vi "main.vi"() -> ()   [LabVIEW 2018]
panel:
  out "First Measurment":bool
  in  "Outfile Path 2":path
  in  "Inital List":string[](array[string])
  in  "Tab Control":T1(tab)
  in  "Sampling Time (s)":u32=2
  in  "Save\n Waveform":bool
  out "Wire Length (mm)":dbl
  out "Linear Density (µg/mm)":dbl
  in  "Save FFT":bool
  in  "sMDT Code":string
  in  "Charge Time (s)":dbl=1.0
  out "Waveform":waveform(dbl)(graph)
  out "FFT":waveform(dbl)(graph)
  out "Charge time(s)":dbl caption="Elapsed Time (s)"
  out "Nth Measurement":i32
  out "DAQ Output (V)":dbl
  out "Tension (g)":dbl format="%#.2f"
  out "Frequency(Hz)":dbl
  in  "User ID":i32(ring) items=["Kyle", "Henry", "Victor", "Dravin", "Braden", "Jake", "Jason", "Akshit", "Jaime", "Mike"]
  out "Charging ?":bool
  in  "Get Tension":bool
  out "Tension Error (g)":dbl format="%#.2g"
  out "Wire Length (mm)":dbl
  out "Linear Density (µg/mm)":dbl
  in  "File Format":enum32{"BMP", "EPS", "EMF", "PICT"}(ring)
  in  "Save Live \nWaveform":bool
  in  "File Format":enum32{"BMP", "EPS", "EMF", "PICT"}(ring)
  out "Live \nWaveform":waveform(dbl)(graph)
  in  "Save Live FFT":bool
  in  "File Format":enum32{"BMP", "EPS", "EMF", "PICT"}(ring)
  out "Live FFT":waveform(dbl)(graph)
  in  "Save Last \nWaveform":bool
  in  "File Format":enum32{"BMP", "EPS", "EMF", "PICT"}(ring)
  out "Last \nWaveform":waveform(dbl)(graph)
  in  "Save Last FFT":bool
  in  "File Format":enum32{"BMP", "EPS", "EMF", "PICT"}(ring)
  out "Last FFT":waveform(dbl)(graph)
  out "Measurements":string[][](array[string])
  in  "Calibration Factor":dbl=1.0
  in  "Frequency Error (Hz)":dbl
  in  "Wire Linear Density Error (µg/mm)":dbl=0.05
  in  "Wire Length Error (mm)":dbl=0.1
  out "User List":string[](array[string])
  in  "Remove":bool
  in  "Add":bool
  in  "User ID":string
  in  "User List File":path
  in  "Wire Linear Density (µg/mm)":dbl=38.8
  # "ATLAS Phase II sMDT Wire Tension Test"
  # "User Controls"
  # "Status"
  # "sMDT Length"
  # "Waveform From Wire"
  # "Measurements"
  # "Spectral Decomposition (FFT)"
  # "Live Wavefrom from Wire"
  # "Live Spectral Decomposition (FFT)"
  # "Last Wavefrom from Wire"
  # "Last Spectral Decomposition (FFT)"
  # "Measurements"
  # "User ID"
  # "Date / Time"
  # "sMDT Code"
  # "Wire Length"
  # "Linear Density"
  # "Frequency"
  # "Tension/g"
  # "Tension/g Error"
  # "Add/Remove Users"
  # "Set Physical Constants"
  # "Calibration"
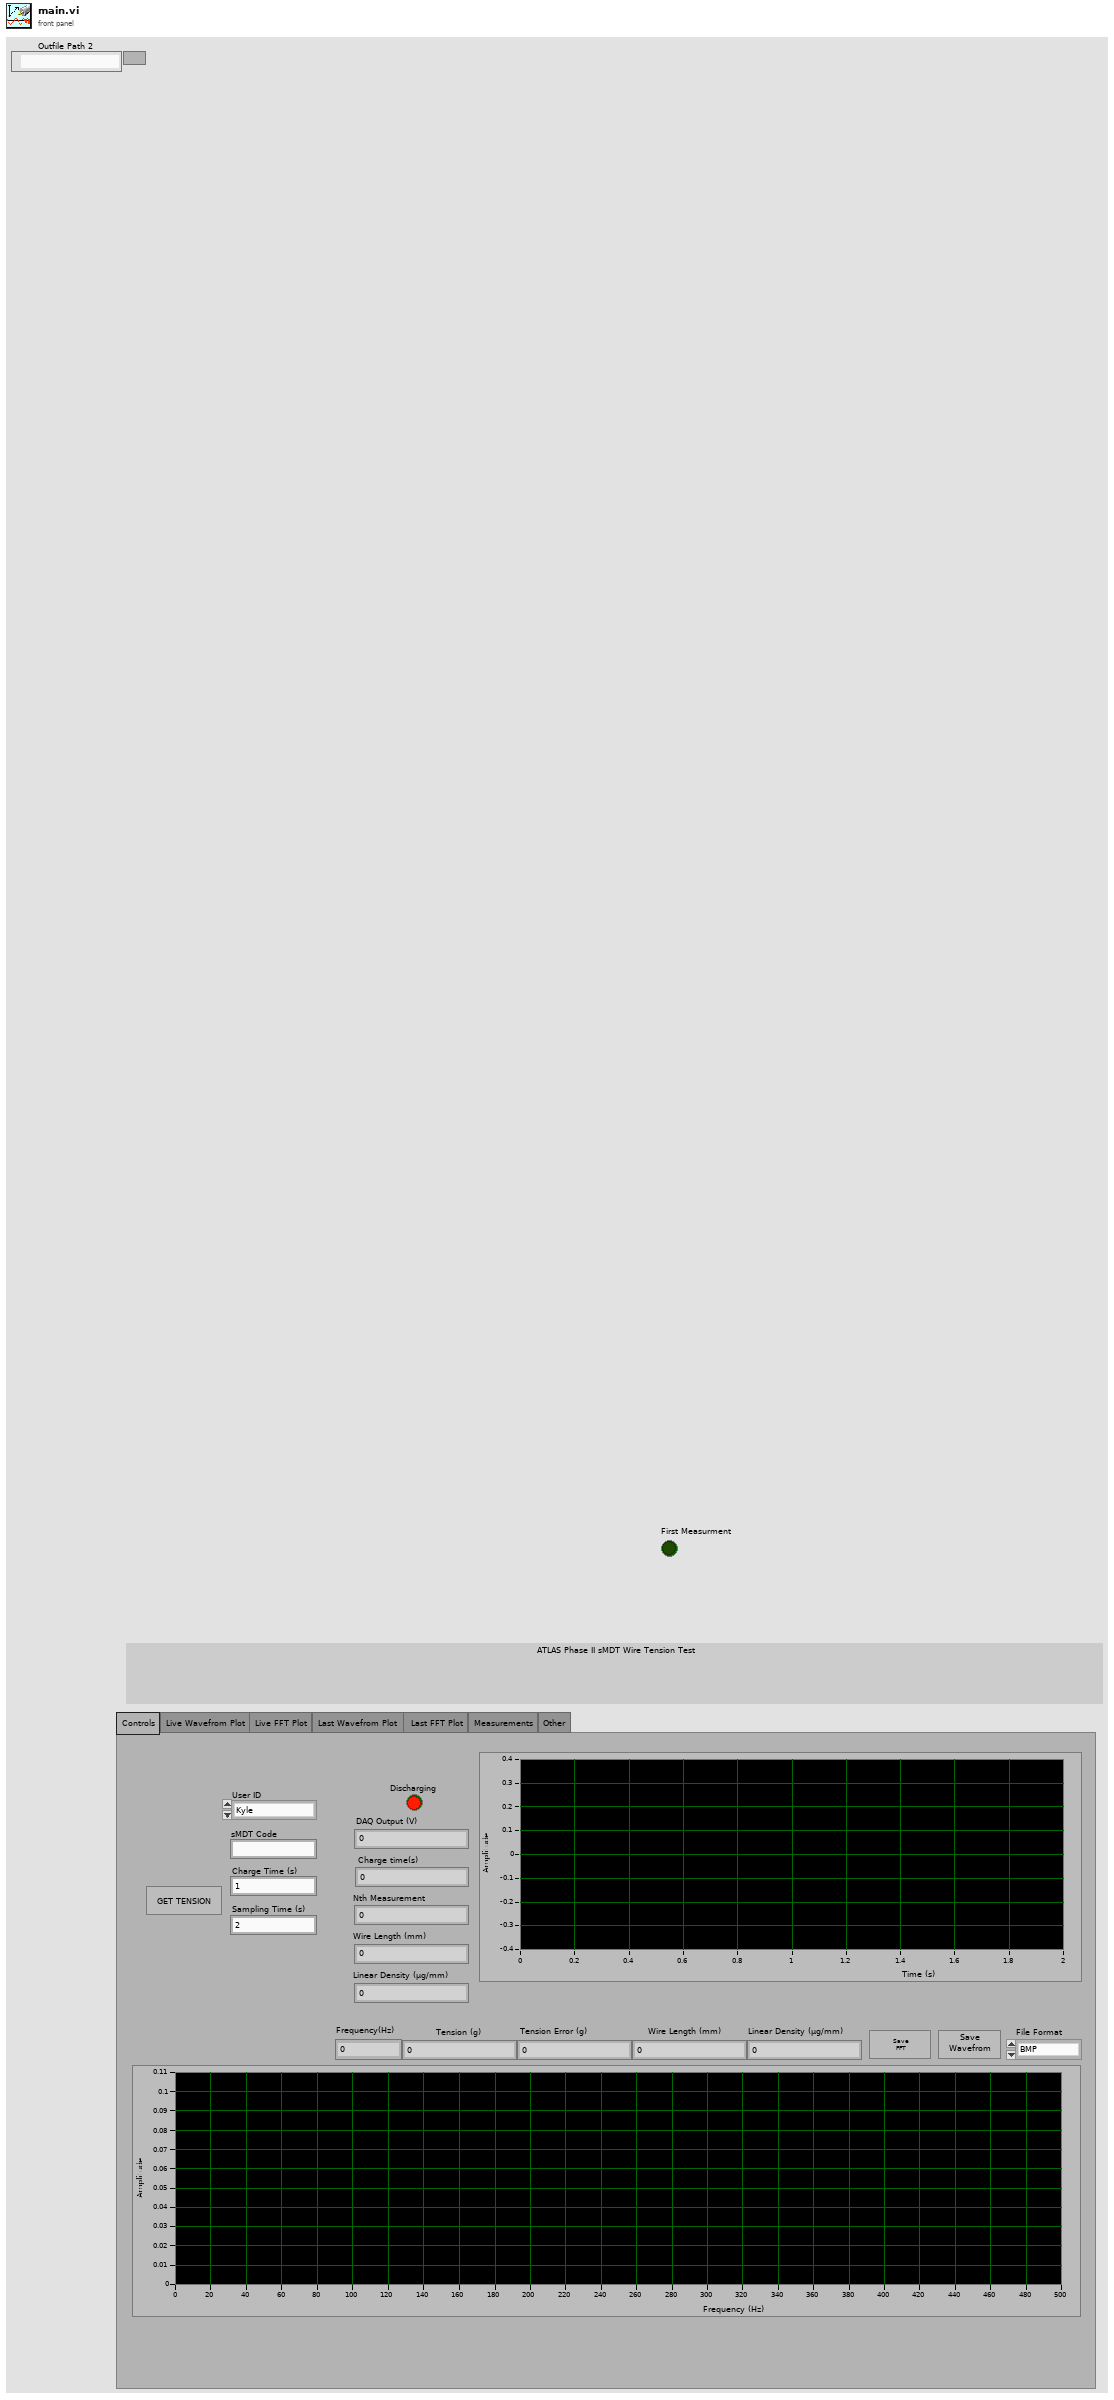
[diagram p1: front panel]
types:
  T1 = enum32{"Controls", "Live Wavefrom Plot", "Live FFT Plot", "Last Wavefrom Plot ", "Last FFT Plot ", "Measurements", "Other"}
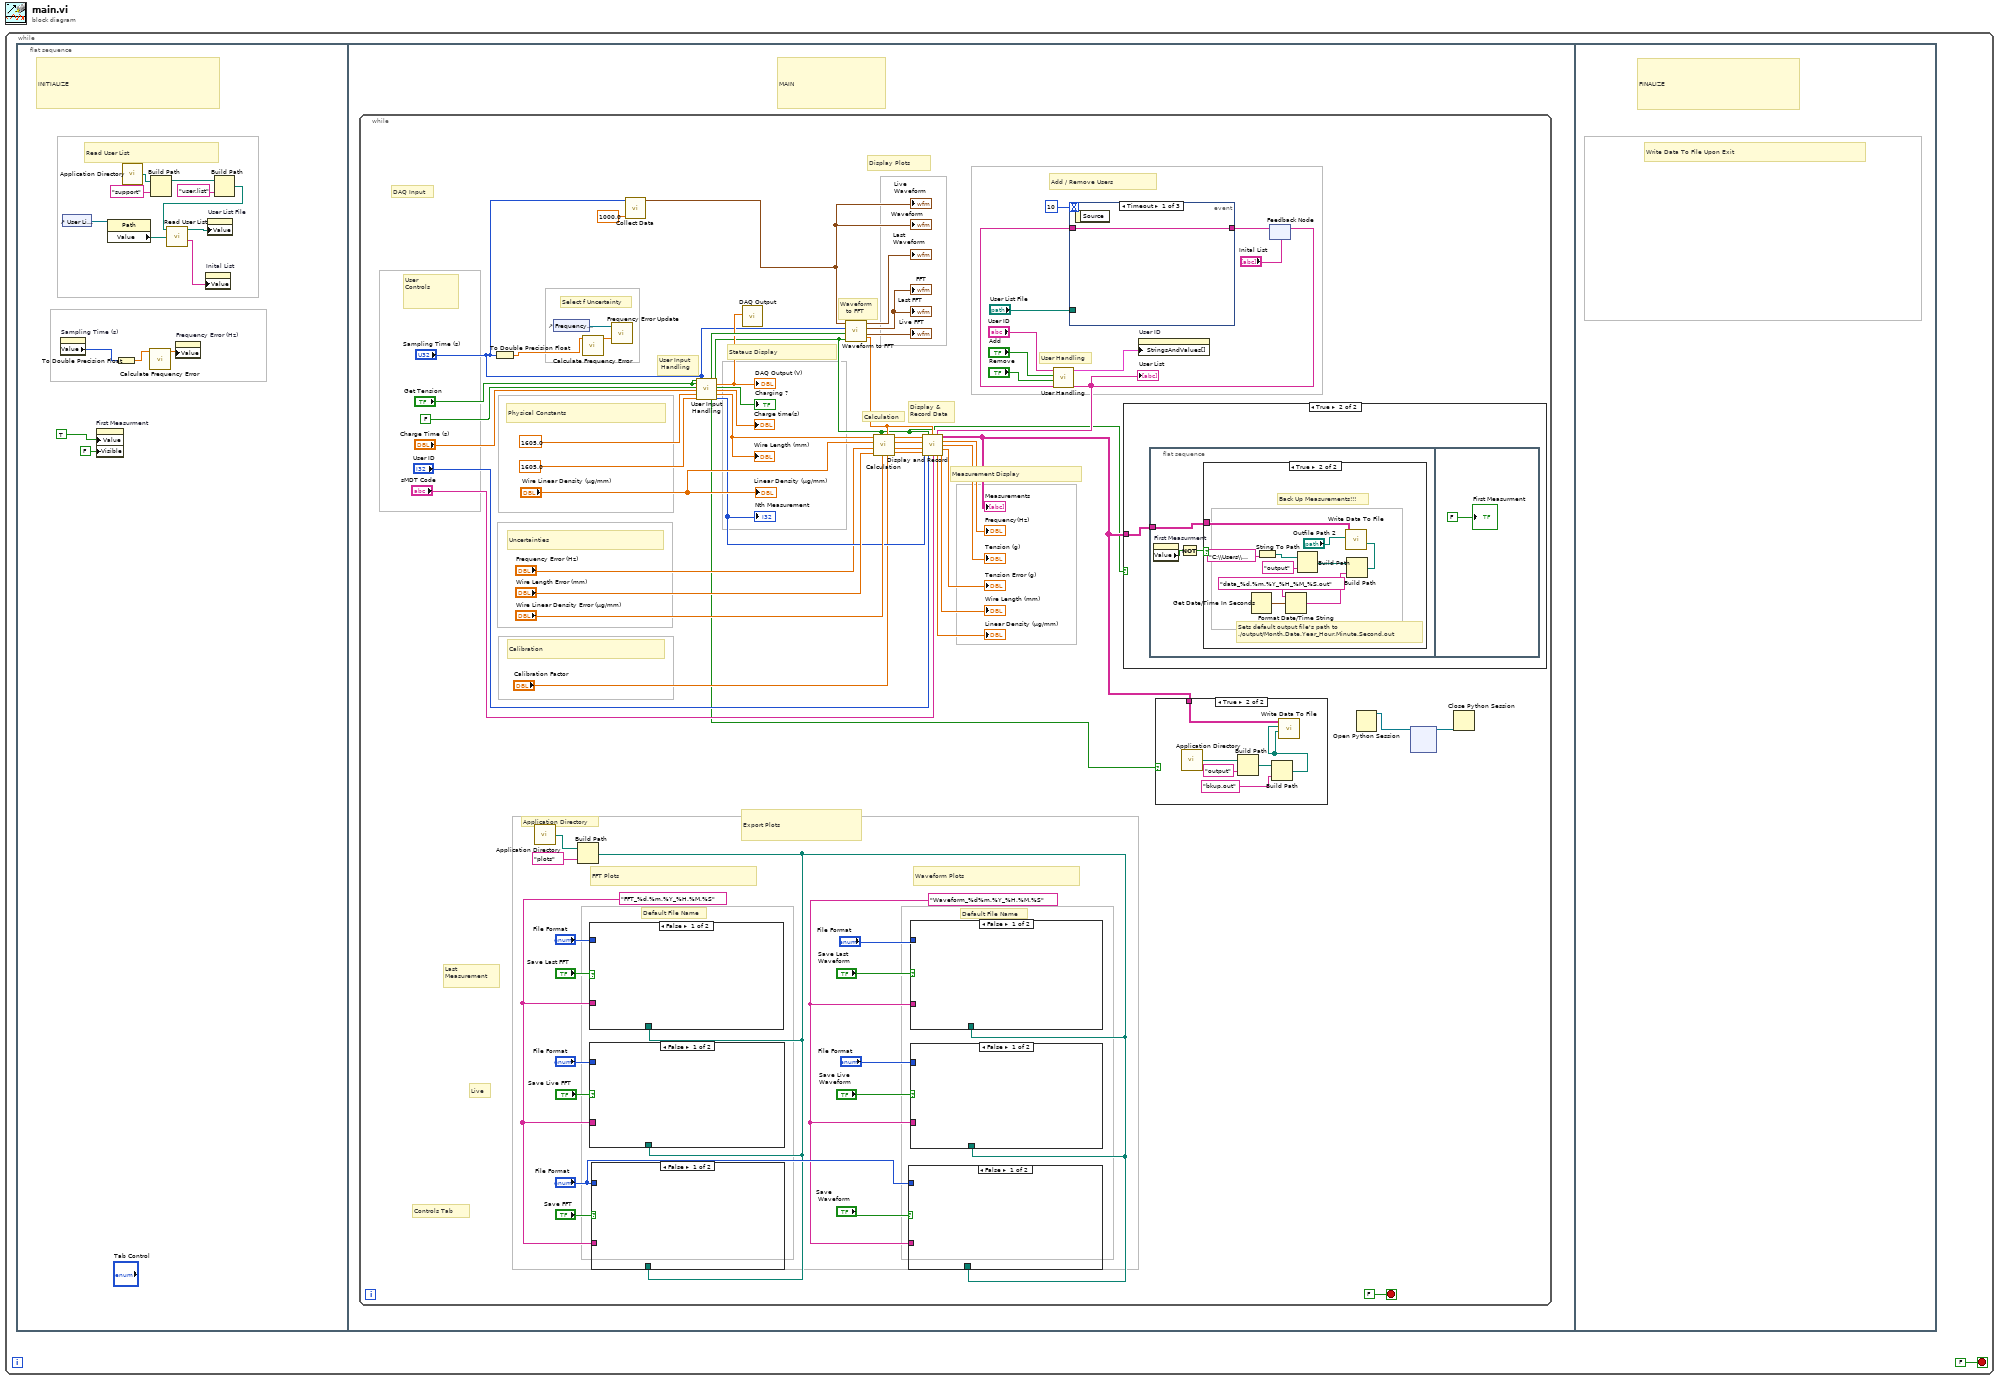
[diagram p0: block diagram]
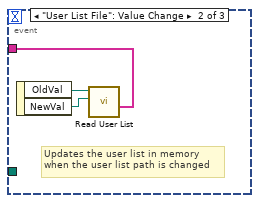
[diagram p5: hidden frame]
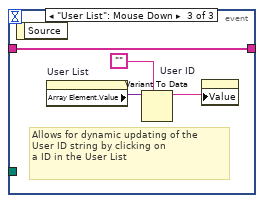
[diagram p6: hidden frame]
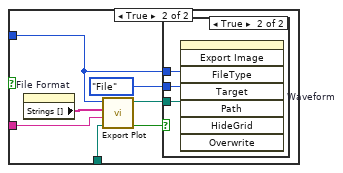
[diagram p7: hidden frame]
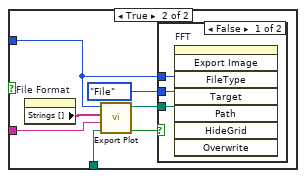
[diagram p9: hidden frame]
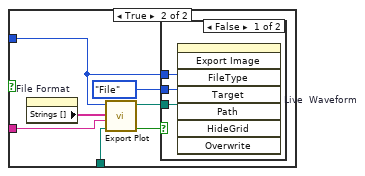
[diagram p11: hidden frame]
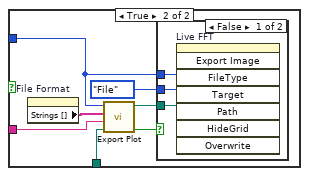
[diagram p13: hidden frame]
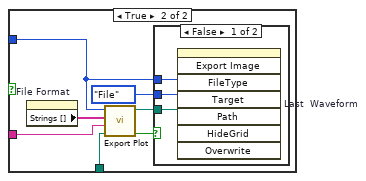
[diagram p15: hidden frame]
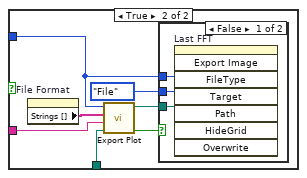
[diagram p17: hidden frame]
diagram:
  n1 = while {
    stop <- FALSE stop-if-true
    n2 = flat-sequence {
      frame #0 {
        # "INITIALIZE"
        # "Read User List"
        n3 = property on="Sampling Time (s)" class="DigNum (strict)"() -> ("Value"=w6:u32)  [unwired: 2 in, 2 out]
        n4 = control-ref of="User List File"() -> (w8:refnum<vi>)
        n5 = property on="First Measurment" class="Bool (strict)"("Value"=TRUE ("First Measurment"), "Visible"=FALSE) -> ()  [unwired: 2 in, 2 out]
        n6 = property on="Property Node" class="Path"(reference=w8) -> ("Value"=w14:path)  [unwired: 1 in, 2 out]
        n7 = To Double Precision Float(number=w6) -> (double precision float=w4:dbl)
        n8 = call <vilib>:"Application Directory.vi"() -> ("Application Directory"=w10:path)
        n9 = call "Calculate Frequency Error.vi"("Sampling Time"=w4) -> ("df"=w5:dbl)  [unwired: 10 in]
        n10 = Build Path(base path=w10, name or relative path="support") -> (appended path=w13:path)
        n11 = property on="Frequency Error (Hz)" class="DigNum (strict)"("Value"=w5) -> ()  [unwired: 2 in, 2 out]
        n12 = Build Path(base path=w13, name or relative path="user.list") -> (appended path=w15:path)
        n13 = call "Read User List.vi"("User List File"=w14, "User List File Default"=w15) -> ("Array"=w9:string[], "Path Out"=w7:path)  [unwired: 8 in]
        n14 = property on="Inital List" class="Arr (strict)"("Value"=w9) -> ()  [unwired: 2 in, 2 out]
        n15 = property on="User List File" class="Path"("Value"=w7) -> ()  [unwired: 2 in, 2 out]
      }
      frame #1 {
        # "MAIN"
        n16 = while {
          stop <- FALSE stop-if-true
          w63 = "Waveform_%d%m.%Y_%H.%M.%S"
          w64 = "FFT_%d.%m.%Y_%H.%M.%S"
          # "User Handling"
          # "Calibration"
          # "Select f Uncertainty"
          # "User Input \n Handling"
          # "Export Plots"
          # "Controls Tab"
          # "Live"
          # "Last \nMeasurement"
          # "Application Directory"
          # "Display Plots"
          # "Default File Name"
          # "Default File Name"
          # "DAQ Input"
          # "Measurement Display"
          # "Stataus Display"
          # "Display &\nRecord Data"
          # "Calculation"
          # "Waveform\n   to FFT"
          # "Waveform Plots"
          # "Uncertainties"
          # "Physical Constants"
          # "FFT Plots"
          # "Add / Remove Users"
          # "User \nControls"
          n17 = To Double Precision Float(number="Sampling Time (s)") -> (double precision float=w30:dbl)
          n18 = call <vilib>:"Application Directory.vi"() -> ("Application Directory"=w35:path)
          n19 = control-ref of="Frequency Error (Hz)"() -> (w37:refnum<vi>)
          n20 = Build Path(base path=w35, name or relative path="plots") -> (appended path=w34:path)
          n21 = call "Calculate Frequency Error.vi"("Sampling Time"=w30) -> ("df"=w31:dbl)  [unwired: 10 in]
          n22 = case shown="False" "Save Last FFT" {
            tunnel: "File Format" -> [_ w164]
            tunnel: w64 -> [_ w170]
            tunnel: w34 -> [_ w169]
            frame False {
            }
            frame True {
              n23 = property on="File Format" class="Enum (strict)"() -> ("Strings []"=w168:string[])  [unwired: 2 in, 2 out]
              n24 = call "Export Plot.vi"("Path 2"=w169, "String"=w170, "Array"=w168, "File Format"=w164) -> ("Canceled?"=w167:bool, "Path"=w166:path)  [unwired: 6 in]
              n25 = case shown="False" w167 {
                tunnel: w166 -> [w173 _]
                tunnel: enum32{"File", "Clipboard"}."File" ("Target") -> [w172 _]
                tunnel: w164 -> [w171 _]
                frame False {
                  n26 = invoke on="Last FFT" class="WFGraph (strict)" method="Export Image"("FileType"=w171, "Target"=w172, "Path"=w173) -> ()  [unwired: 5 in, 8 out]
                }
                frame True {
                }
              }
            }
          }
          n27 = case shown="False" "Save Live FFT" {
            tunnel: w64 -> [_ w150]
            tunnel: w34 -> [_ w149]
            tunnel: "File Format" -> [_ w146]
            frame False {
            }
            frame True {
              n28 = property on="File Format" class="Enum (strict)"() -> ("Strings []"=w145:string[])  [unwired: 2 in, 2 out]
              n29 = call "Export Plot.vi"("Path 2"=w149, "String"=w150, "Array"=w145, "File Format"=w146) -> ("Canceled?"=w144:bool, "Path"=w148:path)  [unwired: 6 in]
              n30 = case shown="False" w144 {
                tunnel: w148 -> [w153 _]
                tunnel: enum32{"File", "Clipboard"}."File" ("Target") -> [w152 _]
                tunnel: w146 -> [w151 _]
                frame False {
                  n31 = invoke on="Live FFT" class="WFGraph (strict)" method="Export Image"("FileType"=w151, "Target"=w152, "Path"=w153) -> ()  [unwired: 5 in, 8 out]
                }
                frame True {
                }
              }
            }
          }
          n32 = case shown="False" "Save FFT" {
            tunnel: "File Format" -> [_ w126]
            tunnel: w64 -> [_ w130]
            tunnel: w34 -> [_ w129]
            frame False {
            }
            frame True {
              n33 = property on="File Format" class="Enum (strict)"() -> ("Strings []"=w125:string[])  [unwired: 2 in, 2 out]
              n34 = call "Export Plot.vi"("Path 2"=w129, "String"=w130, "Array"=w125, "File Format"=w126) -> ("Canceled?"=w124:bool, "Path"=w128:path)  [unwired: 6 in]
              n35 = case shown="False" w124 {
                tunnel: w128 -> [w133 _]
                tunnel: enum32{"File", "Clipboard"}."File" ("Target") -> [w132 _]
                tunnel: w126 -> [w131 _]
                frame False {
                  n36 = invoke on="FFT" class="WFGraph (strict)" method="Export Image"("FileType"=w131, "Target"=w132, "Path"=w133) -> ()  [unwired: 5 in, 8 out]
                }
                frame True {
                }
              }
            }
          }
          n37 = call "Frequency Error Update.vi"("Source"=w31, "Target"=w37) -> ()  [unwired: 10 in]
          n38 = call "Collect Data.vi"("rate"=1000.0, "sample time"="Sampling Time (s)") -> ("Waveform"=w28:waveform(dbl))  [unwired: 9 in]
          "Waveform" <- w28
          "Live \nWaveform" <- w28
          n39 = call "User Input Handling.vi"("Record?"="Get Tension", "Get Tension"="Get Tension", "Short"=FALSE, "Charge Time (s)"="Charge Time (s)", "Short Wire Length (mm)"=1605.0, "Long Wire Length (mm)"=1605.0, "Sampling Time (s)"="Sampling Time (s)") -> ("Has measured?"=w48:bool, "Made Measurement?"=w22:bool, "t < X ?"=w18:bool, "DAQ"=w29:dbl, "charging"=→"Charging ?":bool, "Elapsed time(s)"=→"Charge time(s)":dbl, "Wire Length Out"=w54:dbl, "Nth Measurement"=w49:i32)  [unwired: 5 in]
          "Nth Measurement" <- w49
          "DAQ Output (V)" <- w29
          "Wire Length (mm)" <- w54
          n40 = call "DAQ Output.vi"("Numeric"=w29) -> ()  [unwired: 11 in]
          n41 = call "Waveform to FFT.vi"("t < X ?"=w18, "Measured?"=w48, "Sampling Time(s)"="Sampling Time (s)", "Waveform in"=w28) -> ("FFT out"=→"Live FFT":waveform(dbl), "Last FFT"=→"FFT" →"Last FFT":waveform(dbl), "Last Waveform"=→"Last \nWaveform":waveform(dbl), "Frequency"=w62:dbl)  [unwired: 4 in]
          n42 = call "Calculation.vi"("Calibration Factor"="Calibration Factor", "Frequency (Hz)"=w62, "dµ (µg/mm)"="Wire Linear Density Error (µg/mm)", "t < 1.5 s ?"=w18, "dL (mm)"="Wire Length Error (mm)", "df (Hz)"="Frequency Error (Hz)", "Wire Linear Density In"="Wire Linear Density (µg/mm)", "Wire Length In"=w54) -> ("Linear Density (µm/mm)"=w77:dbl, "Wire Length (mm)"=w76:dbl, "dT (g)"=w75:dbl, "Tension (g)"=w78:dbl)
          n43 = case shown="False" "Save\n Waveform" {
            tunnel: "File Format" -> [_ w117]
            tunnel: w63 -> [_ w120]
            tunnel: w34 -> [_ w119]
            frame False {
            }
            frame True {
              n44 = property on="File Format" class="Enum (strict)"() -> ("Strings []"=w115:string[])  [unwired: 2 in, 2 out]
              n45 = call "Export Plot.vi"("Path 2"=w119, "String"=w120, "Array"=w115, "File Format"=w117) -> ("Canceled?"=w114:bool, "Path"=w118:path)  [unwired: 6 in]
              n46 = case shown="True" w114 {
                tunnel: w118 -> [_ w123]
                tunnel: w117 -> [_ w122]
                tunnel: enum32{"File", "Clipboard"}."File" ("Target") -> [_ w121]
                frame False {
                }
                frame True {
                  n47 = invoke on="Waveform" class="WFGraph (strict)" method="Export Image"("FileType"=w122, "Target"=w121, "Path"=w123) -> ()  [unwired: 5 in, 8 out]
                }
              }
            }
          }
          n48 = case shown="False" "Save Last \nWaveform" {
            tunnel: "File Format" -> [_ w156]
            tunnel: w63 -> [_ w160]
            tunnel: w34 -> [_ w159]
            frame False {
            }
            frame True {
              n49 = property on="File Format" class="Enum (strict)"() -> ("Strings []"=w155:string[])  [unwired: 2 in, 2 out]
              n50 = call "Export Plot.vi"("Path 2"=w159, "String"=w160, "Array"=w155, "File Format"=w156) -> ("Canceled?"=w154:bool, "Path"=w158:path)  [unwired: 6 in]
              n51 = case shown="False" w154 {
                tunnel: w158 -> [w163 _]
                tunnel: enum32{"File", "Clipboard"}."File" ("Target") -> [w162 _]
                tunnel: w156 -> [w161 _]
                frame False {
                  n52 = invoke on="Last  Waveform" class="WFGraph (strict)" method="Export Image"("FileType"=w161, "Target"=w162, "Path"=w163) -> ()  [unwired: 5 in, 8 out]
                }
                frame True {
                }
              }
            }
          }
          n53 = case shown="False" "Save Live \nWaveform" {
            tunnel: w63 -> [_ w140]
            tunnel: "File Format" -> [_ w137]
            tunnel: w34 -> [_ w135]
            frame False {
            }
            frame True {
              n54 = property on="File Format" class="Enum (strict)"() -> ("Strings []"=w136:string[])  [unwired: 2 in, 2 out]
              n55 = call "Export Plot.vi"("Path 2"=w135, "String"=w140, "Array"=w136, "File Format"=w137) -> ("Canceled?"=w134:bool, "Path"=w138:path)  [unwired: 6 in]
              n56 = case shown="False" w134 {
                tunnel: enum32{"File", "Clipboard"}."File" ("Target") -> [w143 _]
                tunnel: w138 -> [w142 _]
                tunnel: w137 -> [w141 _]
                frame False {
                  n57 = invoke on="Live  Waveform" class="WFGraph (strict)" method="Export Image"("FileType"=w141, "Target"=w143, "Path"=w142) -> ()  [unwired: 5 in, 8 out]
                }
                frame True {
                }
              }
            }
          }
          n58 = feedback #1("Inital List") -> (w38:string[])
          n59 = event shown="[0] Timeout" {
            selector: _ -> [_ _ _]
            dyn-events: _ -> [_ _ _]
            timeout: 10 -> [_ _ _]
            tunnel: [w106 w107 w110] -> w45
            tunnel: w38 -> [w106 _ w110]
            tunnel: "User List File" -> [_ _ _]
            event Timeout {
              n60 = event-data() -> ()  [unwired: 1 in, 1 out]
            }
            event "User List File": Value Change {
              # "Updates the user list in memory\nwhen the user list path is changed"
              n61 = event-data() -> ("OldVal"=w109:path, "NewVal"=w108:path)  [unwired: 1 in]
              n62 = call "Read User List.vi"("User List File"=w108, "User List File Default"=w109) -> ("Array"=w107:string[])  [unwired: 8 in, 1 out]
            }
            event "User List": Mouse Down {
              # "Allows for dynamic updating of the \nUser ID string by clicking on \na ID in the User List"
              n63 = event-data() -> ()  [unwired: 1 in, 1 out]
              n64 = property on="User List" class="Arr (strict)"() -> ("Array Element.Value"=w111:variant)  [unwired: 2 in, 2 out]
              n65 = Variant To Data(type="", Variant=w111) -> (data=w112:string)  [unwired: 1 in, 1 out]
              n66 = property on="User ID" class="Str"("Value"=w112) -> ()  [unwired: 2 in, 2 out]
            }
          }
          n67 = call "User Handling.vi"("File In"=w45, "Delete"="Remove", "Add"="Add", "Name"="User ID") -> ("File Out"=w42:string[], "Array"=w84:cluster{"String":string, "Numeric":dbl}[])  [unwired: 4 in]
          "User List" <- w42
          n68 = call "Display and Record.vi"("Tension (g)"=w78, "t < 1.5 s ?"=w18, "Frequency (Hz)"=w62, "User List"=w42, "dT (g)"=w75, "Wire Length (mm)"=w76, "Linear Density (µm/mm)"=w77, "Nth Measurement"=w49, "User ID"="User ID", "sMDT Code"="sMDT Code") -> ("Data Array"=w20:string[][], "Frequency Out"=→"Frequency(Hz)":dbl, "Tension Out"=→"Tension (g)":dbl, "dT Out"=→"Tension Error (g)":dbl, "Linear Density Out"=→"Linear Density (µg/mm)":dbl, "Wire Length Out"=→"Wire Length (mm)":dbl)
          "Measurements" <- w20
          n69 = case shown="True" w18 {
            tunnel: w20 -> [_ w85]
            frame False {
            }
            frame True {
              n70 = flat-sequence {
                tunnel: w85 -> [w88]
                frame #0 {
                  n71 = property on="First Measurment" class="Bool (strict)"() -> ("Value"=w86:bool)  [unwired: 2 in, 2 out]
                  n72 = Not(x=w86) -> (.not. x?=w87:bool)
                  n73 = case shown="True" w87 {
                    tunnel: w88 -> [_ w89]
                    frame False {
                    }
                    frame True {
                      # "Sets default output file's path to \n./output/Month.Date.Year_Hour.Minute.Second.out"
                      # "Back Up Measurements!!!"
                      n74 = Get Date/Time In Seconds() -> (seconds since 1Jan1904=w97:timestamp)
                      n75 = String To Path(string="C:\\Users\\Tension\\Dropbox\\sMDT\\TensionStation") -> (path=w90:path)
                      n76 = Format Date/Time String(time format string (%c)="data_%d.%m.%Y_%H_%M_%S.out", seconds (now)=w97) -> (date/time string=w92:string)  [unwired: 1 in]
                      n77 = Build Path(base path=w90, name or relative path="output") -> (appended path=w94:path)
                      n78 = Build Path(base path=w94, name or relative path=w92) -> (appended path=w95:path)
                      n79 = call "Write Data To File.vi"("Default Path"=w95, "Path"="Outfile Path 2", "Measurements"=w89) -> ()  [unwired: 9 in]
                    }
                  }
                }
                frame #1 {
                  "First Measurment" <- FALSE ("First Measurment")
                }
              }
            }
          }
          n80 = property on="User ID" class="Ring (strict)"("StringsAndValues[]"=w84) -> ()  [unwired: 2 in, 2 out]
          n81 = case shown="True" w22 {
            tunnel: w20 -> [_ w105]
            frame False {
            }
            frame True {
              n82 = call <vilib>:"Application Directory.vi"() -> ("Application Directory"=w103:path)
              n83 = Build Path(base path=w103, name or relative path="output") -> (appended path=w104:path)
              n84 = Build Path(base path=w104, name or relative path="bkup.out") -> (appended path=w101:path)
              n85 = call "Write Data To File.vi"("Default Path"=w101, "Path"=w101, "Measurements"=w105) -> ()  [unwired: 9 in]
            }
          }
          n86 = feedback-in #1(w42) -> ()
          n87 = Open Python Session() -> (session out=w17:refnum<k35>)  [unwired: 3 in, 1 out]
          n88 = node(w17) -> (w16:refnum<k35>)  [unwired: 5 in, 3 out]
          n89 = Close Python Session(session in=w16) -> ()  [unwired: 1 in, 1 out]
          "Linear Density (µg/mm)" <- "Wire Linear Density (µg/mm)"
        }
      }
      frame #2 {
        # "FINALIZE"
        # "Write Data To File Upon Exit"
      }
    }
  }
